vi "Message with Double Quotes.vi"(8 "Error In":errorcluster) -> (0 "Error Out":errorcluster)   [LabVIEW 2018, in "Tests.lvlib"]
uses:
  Tests.lvlib
  src/Toolkit/Support/Manager.vi
  <vilib>/addons/_JKI Toolkits/Caraya/classes/Test/Test.lvclass
  <vilib>/addons/_JKI Toolkits/Caraya/classes/Assert/Assert.lvclass
  src/Toolkit/Toolkit.lvlib
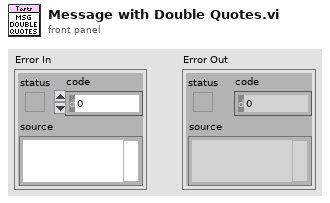
[diagram p1: front panel]
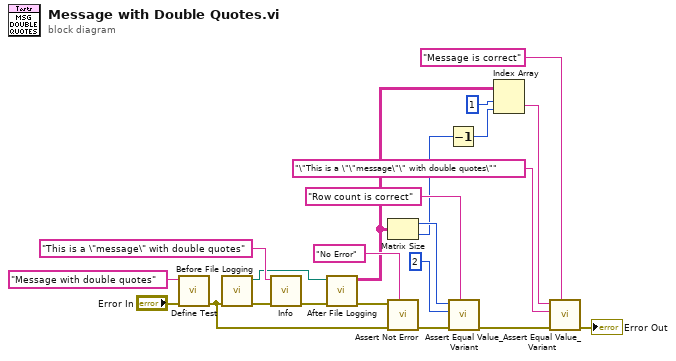
[diagram p0: block diagram]
diagram:
  n1 = call <vilib>:"Define Test.vi"("error in (no error)"="Error In", "Label (VI Title)"="Message with double quotes") -> ("error out"=w1:errorcluster)  [unwired: 9 in]
  n2 = call "Before File Logging.vi"("Error In"=w1) -> ("Error Out"=w19:errorcluster, "Test Log Folder"=w15:path)  [unwired: 9 in]
  n3 = call "Info.vi"("Error In"=w19, "Message"="This is a \"message\" with double quotes") -> ("Error Out"=w18:errorcluster)  [unwired: 9 in]
  n4 = call "After File Logging.vi"("Error In"=w18, "Test Log Folder"=w15) -> ("Error Out"=w2:errorcluster, "Records"=w11:string[][])  [unwired: 8 in]
  n5 = Matrix Size(0:w11) -> (1:w14:i32, 2:w9:i32)
  n6 = call <vilib>:"Assert Not Error.vi"("Label"="No Error", "error in (no error)"=w1, "Not Error?"=w2) -> ("error out"=w16:errorcluster)  [unwired: 8 in]
  n7 = Decrement(x=w9) -> (x-1=w8:i32)
  n8 = call <vilib>:"Assert Equal Value_Variant.vi"("Label"="Row count is correct", "error in (no error)"=w16, "Y"=2 ("size(s)"), "X"=w14) -> ("error out"=w7:errorcluster)  [unwired: 7 in]
  n9 = Index Array(array=w11, index (row)=1, index (col)=w8) -> (element=w3:string)
  n10 = call <vilib>:"Assert Equal Value_Variant.vi"("Label"="Message is correct", "error in (no error)"=w7, "Y"="\"This is a \"\"message\"\" with double quotes\"" ("Message"), "X"=w3) -> ("error out"=→"Error Out":errorcluster)  [unwired: 7 in]
